vi "Read SN.vi"(8 "error in (no error)":errorcluster, 11 "Hitronics in":refnum<class "Hitronics.lvclass">) -> (0 "error out":errorcluster, 3 "Hitronics out":refnum<class "Hitronics.lvclass">)   [LabVIEW 2018, in "Hitronics.lvlib" / "Hitronics.lvclass"]
uses:
  Hitronics.lvclass
  PPLs/Laser/Parent/Laser.lvlibp/Laser.lvclass
  C:/AME Test Engineering/LabVIEW/PPLs/Laser/Parent/Laser.lvlibp/Laser.lvclass
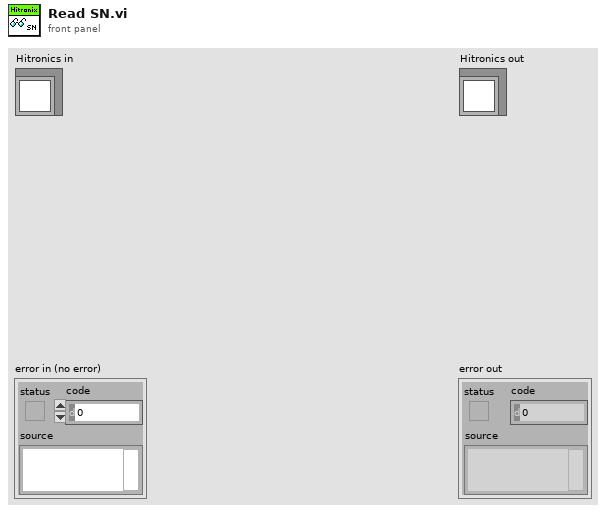
[diagram p1: front panel]
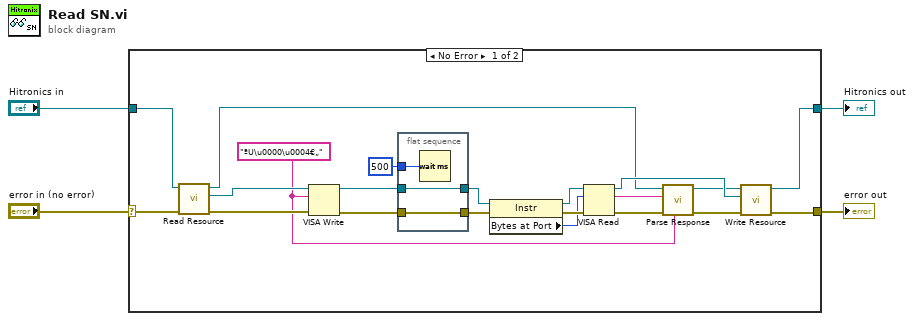
[diagram p0: block diagram]
diagram:
  n1 = case shown="No Error" "error in (no error)" {
    selector: "error in (no error)" -> [w25 w30]
    tunnel: [w11 w30] -> w3
    tunnel: [w12 w29] -> w1
    tunnel: "Hitronics in" -> [w24 w29]
    frame No Error {
      w5 = "ªU\u0000\u0004€„" ("Command")
      n2 = call "Read Resource.vi"("error in (no error)"=w25, "Laser in"=w24) -> ("error out"=w22:errorcluster, "Resource"=w23:refnum<visa-resource-name>, "Laser out"=w6:refnum<class "Hitronics.lvclass">)  [unwired: 7 in]
      n3 = VISA Write(VISA resource name=w23, write buffer=w5, error in (no error)=w22) -> (VISA resource name out=w21:refnum<visa-resource-name>, error out=w20:errorcluster)  [unwired: 1 out]
      n4 = flat-sequence {
        tunnel: w20 -> [w27]
        tunnel: [w27] -> w18
        tunnel: w21 -> [w26]
        tunnel: [w26] -> w17
        tunnel: u32 500 ("delay before read (ms)") -> [w28]
        frame #0 {
          n5 = Wait (ms)(milliseconds to wait=w28) -> ()  [unwired: 1 out]
        }
      }
      n6 = property class="Instr"(reference=w17, error in=w18) -> (reference out=w15:refnum<visa-resource-name>, error out=w16:errorcluster, "Bytes at Port"=w14:u32)
      n7 = VISA Read(VISA resource name=w15, byte count=w14, error in (no error)=w16) -> (VISA resource name out=w13:refnum<visa-resource-name>, read buffer=w10:string, error out=w9:errorcluster)  [unwired: 1 out]
      n8 = call "Parse Response.vi"("Command String (Hex)"=w5, "error in (no error)"=w9, "Response String (Hex)"=w10, "Hitronics in"=w6) -> ("error out"=w8:errorcluster, "Hitronics out"=w7:refnum<class "Hitronics.lvclass">)  [unwired: 5 in, 1 out]
      n9 = call "Write Resource.vi"("error in (no error)"=w8, "Resource"=w13, "Laser in"=w7) -> ("error out"=w11:errorcluster, "Laser out"=w12:refnum<class "Hitronics.lvclass">)  [unwired: 7 in]
    }
    frame Error {
    }
  }
  "error out" <- w3
  "Hitronics out" <- w1
